vi "ECM_Lambda_Propane.vi"(8 "V In":dbl) -> (0 "Lambda Propene":dbl, 1 "Lambda Corr":dbl, 2 "Lambda Gasoline":dbl)   [LabVIEW 2014]
panel:
  out "AFR Gasoline":dbl
  out "AFR Corr":dbl
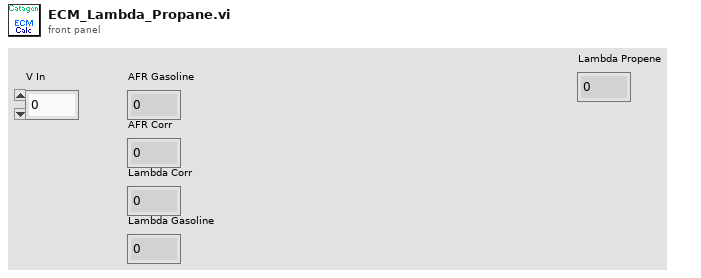
[diagram p1: front panel]
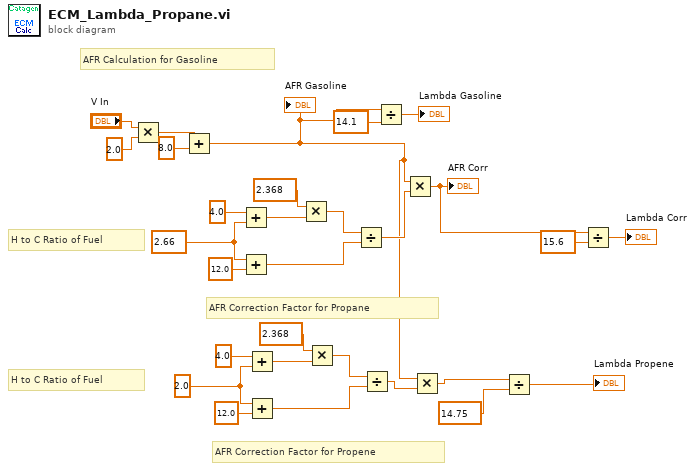
[diagram p0: block diagram]
diagram:
  w9 = 2.0 ("y")
  w24 = 2.66 ("y")
  # "H to C Ratio of Fuel"
  # "AFR Correction Factor for Propene"
  # "H to C Ratio of Fuel"
  # "AFR Correction Factor for Propane"
  # "AFR Calculation for Gasoline"
  n1 = Multiply(x="V In", y=2.0) -> (x*y=w20:dbl)
  n2 = Add(x=w20, y=8.0) -> (x+y=w4:dbl)
  "AFR Gasoline" <- w4
  n3 = Add(x=4.0 ("y"), y=w24) -> (x+y=w26:dbl)
  n4 = Add(x=w24, y=12.0) -> (x+y=w21:dbl)
  n5 = Add(x=4.0 ("y"), y=w9) -> (x+y=w7:dbl)
  n6 = Add(x=w9, y=12.0) -> (x+y=w12:dbl)
  n7 = Multiply(x=2.368, y=w26) -> (x*y=w22:dbl)
  n8 = Multiply(x=2.368, y=w7) -> (x*y=w11:dbl)
  n9 = Divide(x=w22, y=w21) -> (x/y=w18:dbl)
  n10 = Divide(x=w11, y=w12) -> (x/y=w5:dbl)
  n11 = Divide(x=w4, y=14.1) -> (x/y=→"Lambda Gasoline":dbl)
  n12 = Multiply(x=w4, y=w18) -> (x*y=w17:dbl)
  "AFR Corr" <- w17
  n13 = Multiply(x=w4, y=w5) -> (x*y=w3:dbl)
  n14 = Divide(x=w3, y=14.75) -> (x/y=→"Lambda Propene":dbl)
  n15 = Divide(x=w17, y=15.6) -> (x/y=→"Lambda Corr":dbl)
